vi "SIM_CurrentOutput.vi"(6 "Z Write?":bool, 9 "array":dbl[][](array[numeric]), 11 "Position":cluster{"X":dbl, "Y":dbl, "Z pen":dbl, "Z":dbl}) -> (3 "Current Out (pA)":dbl)   [LabVIEW 2017]
uses:
  <vilib>/ptbypt/NI_PtbyPt.lvlib
  GlobalClicksHeight.vi
panel:
  out "Zread":dbl
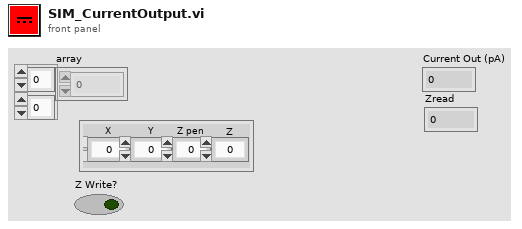
[diagram p1: front panel]
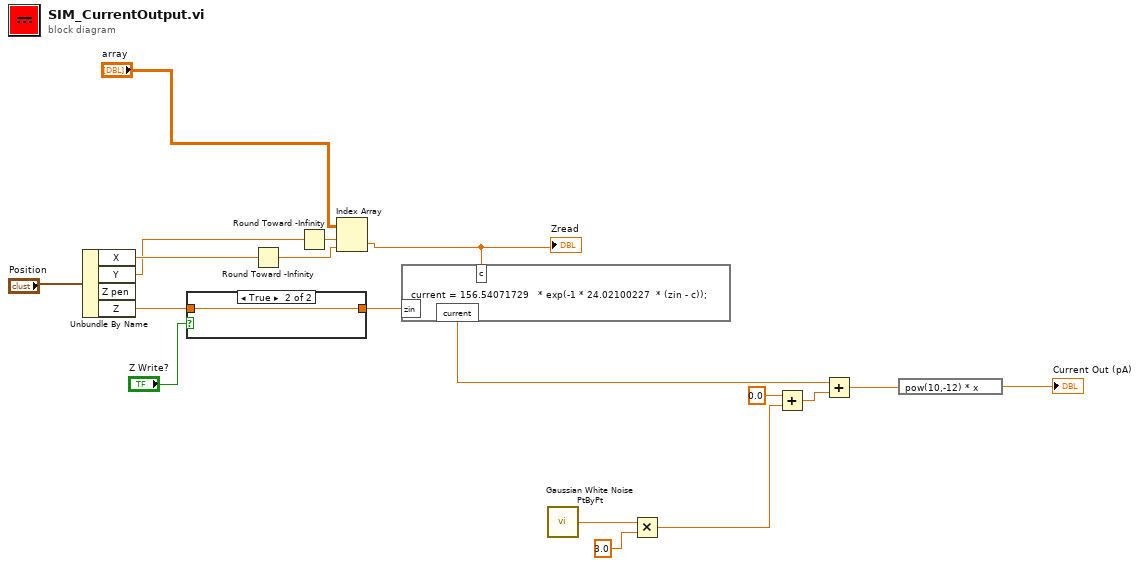
[diagram p0: block diagram]
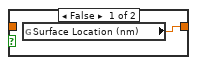
[diagram p2: hidden frame]
diagram:
  n1 = Unbundle By Name("Position") -> ("X"=w8:dbl, "Y"=w7:dbl, "Z"=w2:dbl)  [unwired: 1 out]
  n2 = case shown="True" "Z Write?" {
    tunnel: w2 -> [_ w20]
    tunnel: [w19 w20] -> w1
    frame False {
      n3 = global read "GlobalClicksHeight.vi" "Surface Location (nm)"() -> (w19:dbl)
    }
    frame True {
    }
  }
  n4 = Round Toward -Infinity(1:w8) -> (0:w17:dbl)
  n5 = Round Toward -Infinity(1:w7) -> (0:w18:dbl)
  n6 = Index Array(array="array", index (row)=w18, index (col)=w17) -> (element=w4:dbl)
  "Zread" <- w4
  n7 = formula code="current = 156.54071729   * exp(-1 * 24.02100227  * (zin - c));"("zin"=w1, "c"=w4) -> ("current"=w11:dbl)
  n8 = call <vilib>:"Gaussian White Noise PtByPt.vi"() -> ("Gaussian white noise"=w16:dbl)  [unwired: 3 in]
  n9 = Multiply(x=w16, y=3.0) -> (x*y=w13:dbl)
  n10 = Add(x=0.0, y=w13) -> (x+y=w14:dbl)
  n11 = Add(x=w11, y=w14) -> (x+y=w6:dbl)
  n12 = expression code="pow(10,-12) * x"(w6) -> (→"Current Out (pA)":dbl)
